vi "DataPacker_Stop.vi"(11 "URGENT STOP! (Dont wait for data to finish sending). Default F":bool) -> ()   [LabVIEW 2018, in "feGEM DataPacker.lvlib"]
uses:
  feGEM DataPacker.lvlib
  DataPacker_Commands.ctl
  DataPacker_Settings.ctl
  GlobalVariables/DataPacker_Global_Stop_Enum.ctl
  <vilib>/Utility/SystemLogging/NI_SystemLogging.lvlib
panel:
  out "# elements in queue":i32
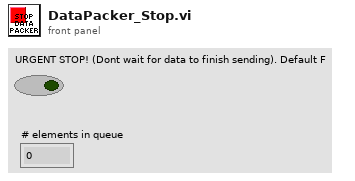
[diagram p1: front panel]
types:
  T1 = typedef "feGEM DataPacker.lvlib/DataPacker_Settings.ctl" = cluster{"Override Max Event size (Data rate kb/s). Use MIDAS Default = 0":u32, "MIDAS Server":string, "MIDAS Server Port":u16, "Max Queue Size (-1, unlimited)":i32, "DataPacker_Command":T2, "Caller VI":string[]}
  T2 = typedef "feGEM DataPacker.lvlib/DataPacker_Commands.ctl" = enum16{"Do Nothing", "Restart", "Stop"}
  T3 = typedef "feGEM DataPacker.lvlib/DataPacker_Global_Stop_Enum.ctl" = enum16{"Reset", "Set Soft Stop", "Get Soft Stop", "Set Hard Stop", "Get Hard Stop", "Get Any Stop"}
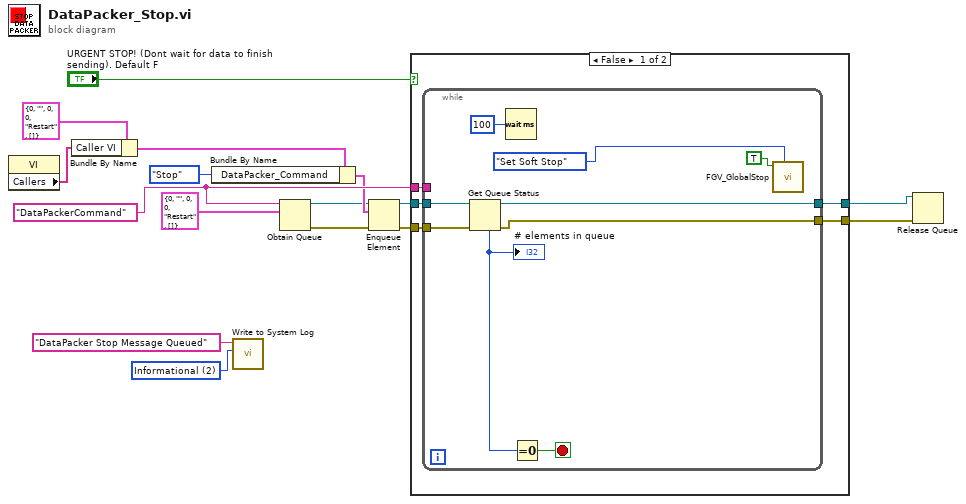
[diagram p0: block diagram]
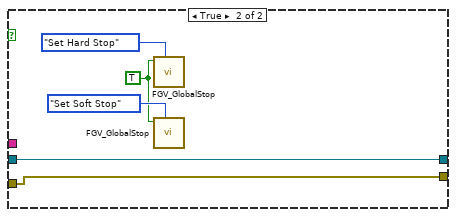
[diagram p2: hidden frame]
diagram:
  w2 = 2 items=["Error", "Warning", "Informational"] ("severity")
  w12 = "DataPackerCommand" ("name (unnamed)")
  n1 = property class="VI"() -> ("Callers"=w16:string[])  [unwired: 2 in, 2 out]
  n2 = Bundle By Name(cluster=T1 {"Override Max Event size (Data rate kb/s). Use MIDAS Default = 0"=0, "MIDAS Server"="", "MIDAS Server Port"=0, "Max Queue Size (-1, unlimited)"=0, "DataPacker_Command"=enum."Restart", "Caller VI"=[]} ("output cluster"), "Caller VI"=w16) -> (w8:T1)
  n3 = Bundle By Name(cluster=w8, "DataPacker_Command"=DataPacker_Commands."Stop") -> (w11:T1)
  n4 = call <vilib>:"Write to System Log.vi"("severity"=w2, "message"="DataPacker Stop Message Queued") -> ()  [unwired: 9 in, 1 out]
  n5 = Obtain Queue(name (unnamed)=w12, element data type=T1 {"Override Max Event size (Data rate kb/s). Use MIDAS Default = 0"=0, "MIDAS Server"="", "MIDAS Server Port"=0, "Max Queue Size (-1, unlimited)"=0, "DataPacker_Command"=enum."Restart", "Caller VI"=[]} ("output cluster")) -> (queue out=w10:refnum<queue>, error out=w9:errorcluster)  [unwired: 3 in, 1 out]
  n6 = Enqueue Element(queue=w10, element=w11, error in (no error)=w9) -> (queue out=w6:refnum<queue>, error out=w5:errorcluster)  [unwired: 1 in, 1 out]
  n7 = case shown="False" "URGENT STOP! (Dont wait for data to finish sending). Default F" {
    tunnel: w12 -> [w21 _]
    tunnel: [w20 w35] -> w4
    tunnel: [w19 w34] -> w3
    tunnel: w6 -> [w18 w35]
    tunnel: w5 -> [w17 w34]
    frame False {
      n8 = while {
        tunnel: w21 -> [_]
        tunnel: [w30] -> w20
        tunnel: [w29] -> w19
        tunnel: w18 -> [w26]
        tunnel: w17 -> [w25]
        stop <- w22 stop-if-true
        n9 = Get Queue Status(queue=w26, error in (no error)=w25) -> (queue out=w30:refnum<queue>, error out=w29:errorcluster, # elements in queue=w28:i32)  [unwired: 1 in, 5 out]
        "# elements in queue" <- w28
        n10 = Wait (ms)(milliseconds to wait=u32 100) -> ()  [unwired: 1 out]
        n11 = Equal To 0?(x=w28) -> (x = 0?=w22:bool)
        n12 = call "FGV_GlobalStop.vi"("Stop"=TRUE, "Enum"=DataPacker_Global_Stop_Enum."Set Soft Stop") -> ()  [unwired: 3 in, 1 out]
      }
    }
    frame True {
      w31 = TRUE ("Stop")
      n13 = call "FGV_GlobalStop.vi"("Stop"=w31, "Enum"=DataPacker_Global_Stop_Enum."Set Hard Stop") -> ()  [unwired: 3 in, 1 out]
      n14 = call "FGV_GlobalStop.vi"("Stop"=w31, "Enum"=DataPacker_Global_Stop_Enum."Set Soft Stop") -> ()  [unwired: 3 in, 1 out]
    }
  }
  n15 = Release Queue(queue=w4, error in (no error)=w3) -> ()  [unwired: 1 in, 3 out]
